vi "Roots_of_2.13_m.vi"(8 "Initialise":bool, 9 "z":dbl format="%.2f", 10 "y*":dbl format="%.2f", 11 "x*":dbl format="%.2f") -> (0 "v":dbl[](array[numeric]) format="%.2f", 1 "u":dbl[](array[numeric]) format="%.2f", 3 "y":dbl[](array[numeric]) format="%.2f", 4 "w":dbl[](array[numeric]) format="%.2f", 5 "x":dbl[](array[numeric]) format="%.2f", 6 "Roots exist":bool)   [LabVIEW 2010]
uses:
  xw_correction_global_m.vi
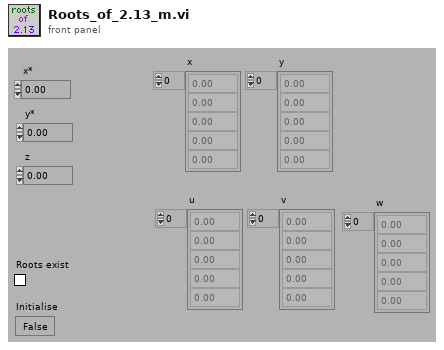
[diagram p1: front panel]
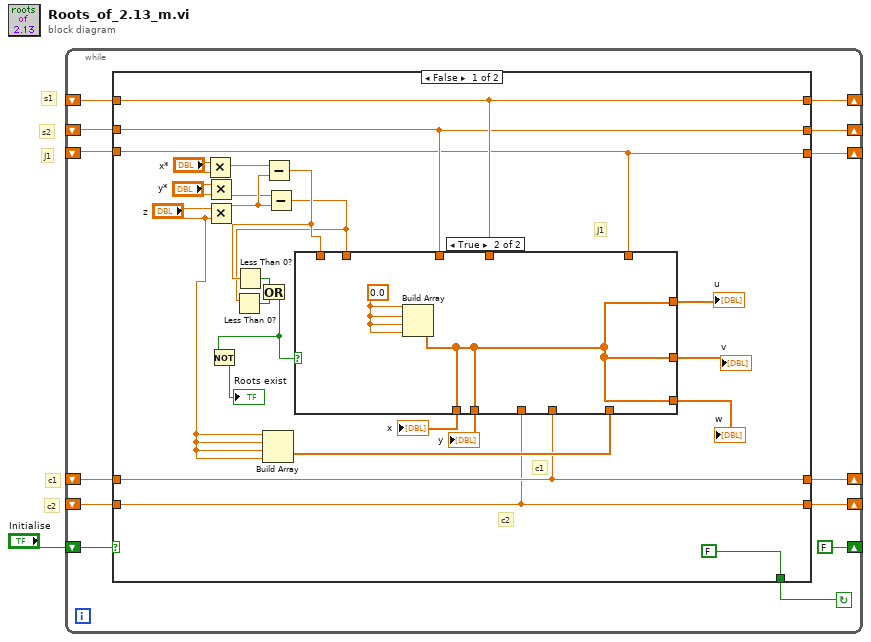
[diagram p0: block diagram]
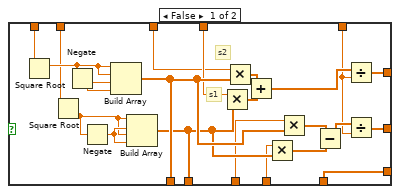
[diagram p2: hidden frame]
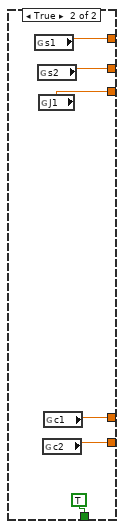
[diagram p3: hidden frame]
diagram:
  # "J1"
  # "s1"
  # "s2"
  # "c2"
  # "c1"
  n1 = while {
    shift-left: _ -> [w3]
    shift-right: [w2] -> _
    shift-left: _ -> [w6]
    shift-right: [w4] -> _
    shift-left: _ -> [w7]
    shift-right: [w5] -> _
    shift-left: _ -> [w10]
    shift-right: [w9] -> _
    shift-left: _ -> [w12]
    shift-right: [w11] -> _
    shift-left: "Initialise" -> [w13]
    shift-right: [FALSE] -> _
    stop <- w14 continue-if-true
    n2 = case shown="False" w13 {
      tunnel: [FALSE TRUE] -> w14
      tunnel: w12 -> [w19 _]
      tunnel: [w19 w68] -> w11
      tunnel: w10 -> [w18 _]
      tunnel: [w18 w67] -> w9
      tunnel: w7 -> [w17 _]
      tunnel: w6 -> [w16 _]
      tunnel: [w17 w64] -> w5
      tunnel: [w16 w65] -> w4
      tunnel: w3 -> [w15 _]
      tunnel: [w15 w63] -> w2
      frame False {
        # "J1"
        # "c2"
        # "c1"
        n3 = Multiply(x="x*", y="x*") -> (x*y=w23:dbl)
        n4 = Multiply(x="y*", y="y*") -> (x*y=w24:dbl)
        n5 = Multiply(x="z", y="z") -> (x*y=w25:dbl)
        n6 = Build Array("z", "z", "z", "z") -> (w26:dbl[])
        n7 = Subtract(x=w23, y=w25) -> (x-y=w22:dbl)
        n8 = Less Than 0?(x=w22) -> (x < 0?=w35:bool)
        n9 = Subtract(x=w24, y=w25) -> (x-y=w21:dbl)
        n10 = Less Than 0?(x=w21) -> (x < 0?=w34:bool)
        n11 = Or(x=w35, y=w34) -> (x .or. y?=w33:bool)
        n12 = Not(x=w33) -> (.not. x?=→"Roots exist":bool)
        n13 = case shown="True" w33 {
          tunnel: w21 -> [w56 _]
          tunnel: w22 -> [w55 _]
          tunnel: [w54 w61] -> w31
          tunnel: [w43 w61] -> w30
          tunnel: [w53 w61] -> w29
          tunnel: w26 -> [w53 _]
          tunnel: [w47 w61] -> w28
          tunnel: [w46 w61] -> w27
          tunnel: w15 -> [w44 _]
          tunnel: w19 -> [w42 _]
          tunnel: w18 -> [w41 _]
          tunnel: w17 -> [w40 _]
          tunnel: w16 -> [w39 _]
          frame False {
            # "s1"
            # "s2"
            n14 = Square Root(x=w55) -> (sqrt(x)=w57:dbl)
            n15 = Square Root(x=w56) -> (sqrt(x)=w59:dbl)
            n16 = Negate(x=w57) -> (-x=w58:dbl)
            n17 = Negate(x=w59) -> (-x=w60:dbl)
            n18 = Build Array(w57, w57, w58, w58) -> (w47:dbl[])
            n19 = Build Array(w59, w60, w59, w60) -> (w46:dbl[])
            n20 = Multiply(x=w40, y=w46) -> (x*y=w51:dbl[])
            n21 = Multiply(x=w39, y=w47) -> (x*y=w52:dbl[])
            n22 = Add(x=w52, y=w51) -> (x+y=w50:dbl[])
            n23 = Multiply(x=w42, y=w46) -> (x*y=w49:dbl[])
            n24 = Multiply(x=w41, y=w47) -> (x*y=w48:dbl[])
            n25 = Subtract(x=w48, y=w49) -> (x-y=w45:dbl[])
            n26 = Divide(x=w50, y=w44) -> (x/y=w54:dbl[])
            n27 = Divide(x=w45, y=w44) -> (x/y=w43:dbl[])
          }
          frame True {
            w62 = 0.0
            n28 = Build Array(w62, w62, w62, w62) -> (w61:dbl[])
          }
        }
        "w" <- w29
        "u" <- w31
        "v" <- w30
        "x" <- w28
        "y" <- w27
      }
      frame True {
        n29 = global read "xw_correction_global_m.vi" "s1"() -> (w64:dbl)
        n30 = global read "xw_correction_global_m.vi" "s2"() -> (w65:dbl)
        n31 = global read "xw_correction_global_m.vi" "J1"() -> (w63:dbl)
        n32 = global read "xw_correction_global_m.vi" "c2"() -> (w67:dbl)
        n33 = global read "xw_correction_global_m.vi" "c1"() -> (w68:dbl)
      }
    }
  }
